vi "Apply Heat.vi"(8 "error in (no error)":errorcluster, 10 "Fire (%)":dbl min=0.0 max=100.0 format="%.2f", 11 "Direct Oven in":refnum<class "Direct Oven.lvclass">) -> (0 "error out":errorcluster, 3 "Direct Oven out":refnum<class "Direct Oven.lvclass">)   [LabVIEW 2024, in "Oven Actor.lvlib" / "Direct Oven.lvclass"]
uses:
  Direct Oven.lvclass
  Direct Oven.lvclass/Direct Oven.ctl
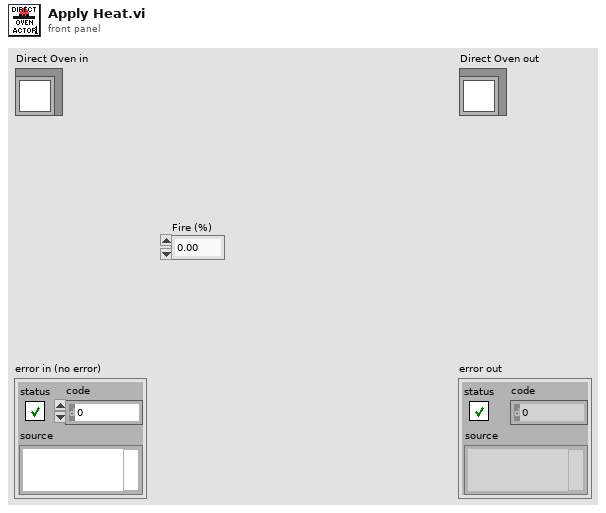
[diagram p1: front panel]
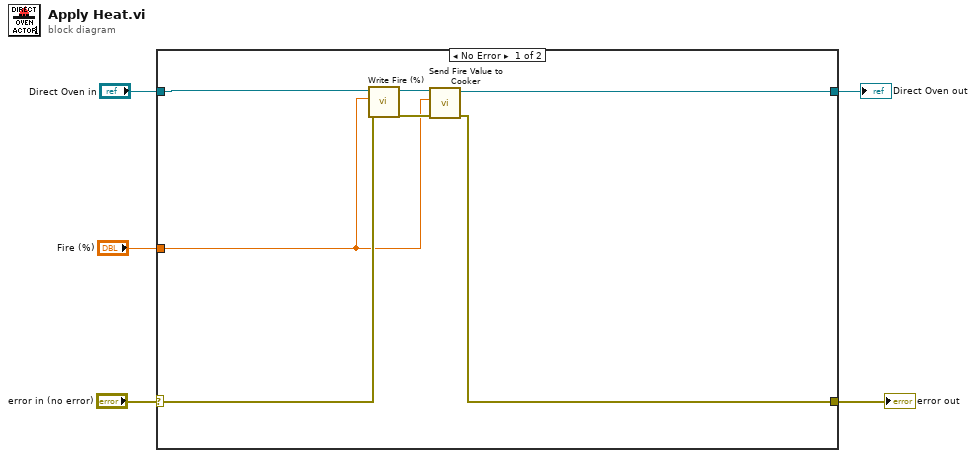
[diagram p0: block diagram]
diagram:
  n1 = case shown="No Error" "error in (no error)" {
    selector: "error in (no error)" -> [w10 w13]
    tunnel: [w12 w13] -> w4
    tunnel: "Direct Oven in" -> [w8 w14]
    tunnel: [w11 w14] -> w2
    tunnel: "Fire (%)" -> [w6 _]
    frame No Error {
      n2 = call-dynamic "Write Fire (%).vi"("error in (no error)"=w10, "Fire (%)"=w6, "Oven Actor in"=w8) -> ("error out"=w9:errorcluster, "Oven Actor out"=w7:refnum<class "Direct Oven.lvclass">)  [unwired: 7 in]
      n3 = call-dynamic "Send Fire Value to Cooker.vi"("error in (no error)"=w9, "Fire (%)"=w6, "Oven Actor in"=w7) -> ("error out"=w12:errorcluster, "Oven Actor out"=w11:refnum<class "Direct Oven.lvclass">)  [unwired: 7 in]
    }
    frame Error {
    }
  }
  "error out" <- w4
  "Direct Oven out" <- w2
